vi "Read Access Time.vi"(8 "Error In":errorcluster, 11 "File Info In":refnum<class "File Info.lvclass">) -> (0 "Error Out":errorcluster, 2 "Access Time":u64, 3 "File Info Out":refnum<class "File Info.lvclass">)   [LabVIEW 2021, in "Field_RnD_Services_LIBSSH2_Toolkit.lvlib" / "File Info.lvclass"]
doc: "Gets the last time the remote filesystem entry was read in seconds relative to the UNIX epoch."
uses:
  220524-VNA RP FLAT.llb/File Info.lvclass
  220524-VNA RP FLAT.llb/File Info.lvclass/File Info.ctl
  220524-VNA RP FLAT.llb/Field_RnD_Services_LIBSSH2_Toolkit.lvlib
  220524-VNA RP FLAT.llb/SSH.lvclass
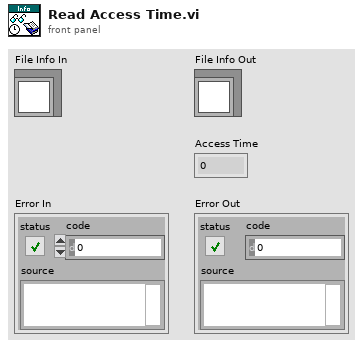
[diagram p1: front panel]
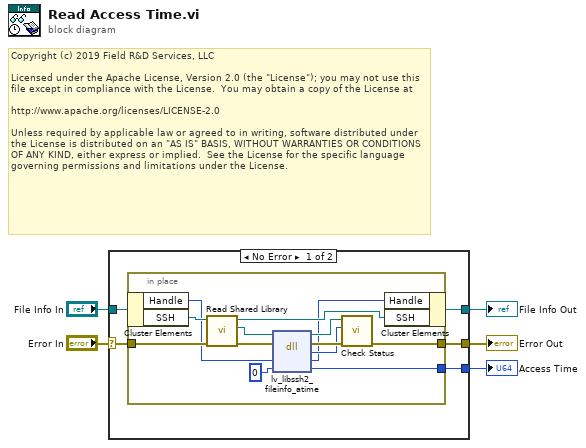
[diagram p0: block diagram]
diagram:
  # "Copyright (c) 2019 Field R&D Services, LLC\n\nLicensed under the Apache License, Version 2.0 (the \"License\"); you may not use this file except in compliance with the License.  You may obtain a copy of the License at\n\nhttp://www.apache.org/licenses/LICENSE-2.0\n\nUnless required by applicable law or agreed to in writing, software distributed under the License is distributed on an \"AS IS\" BASIS, WITHOUT WARRANTIES OR CONDITIONS OF ANY KIND, either express or implied.  See the License for the specific language governing permissions and limitations under the License."
  n1 = case shown="No Error" "Error In" {
    selector: "Error In" -> [w9 w25]
    tunnel: [w7 w25] -> w4
    tunnel: "File Info In" -> [w10 w24]
    tunnel: [w8 w24] -> w2
    tunnel: [w6 _] -> w1
    frame No Error {
      n2 = in-place {
        in-place-border: w9 -> [w16]
        in-place-border: [w13] -> w7
        in-place-border: [w11] -> w6
        n3 = in-place-cluster #1(w10) -> ("Handle"=w15:u64, "SSH"=w20:refnum<class "SSH.lvclass">)
        n4 = call "Read Shared Library.vi"("Error In"=w16, "SSH In"=w20) -> ("Error Out"=w17:errorcluster, "libssh2lv Shared Library"=w18:path, "SSH Out"=w19:refnum<class "SSH.lvclass">)  [unwired: 7 in]
        n5 = dll-call lib="lv-libssh2.*" fn="lv_libssh2_fileinfo_atime"(path in=w18, error in=w17, "handle"=w15, "atime"=u64 0 ("flags")) -> (path out=w22:path, error out=w23:errorcluster, "status"=w21:i32, "handle"=w14:u64, "atime"=w11:u64)  [unwired: 1 in]
        n6 = call "Check Status.vi"("Error In"=w23, "Status"=w21, "libssh2lv Shared Library In"=w22) -> ("Error Out"=w13:errorcluster)  [unwired: 7 in, 1 out]
        n7 = in-place-cluster #1("Handle"=w14, "SSH"=w19) -> (w8:refnum<class "File Info.lvclass">)
      }
    }
    frame Error {
    }
  }
  "Error Out" <- w4
  "File Info Out" <- w2
  "Access Time" <- w1
